vi "captureSpectImage.vi"(8 "error in (no error)":errorcluster, 9 "command_captureSpectImage":T1, 10 "model in":refnum<class "IModel.lvclass">, 11 "DefaultState in":refnum<class "DefaultState.lvclass">) -> (0 "error out":errorcluster, 2 "model out":refnum<class "IModel.lvclass">, 3 "DefaultState out":refnum<class "DefaultState.lvclass">)   [LabVIEW 2016, in "States.lvlib" / "DefaultState.lvclass"]
uses:
  DefaultState.lvclass
  IModel/IModel.lvclass
  ts_sallv_FiberSpectrograph/DataTypes/command_captureSpectImage.ctl
  Typedefs/CommandValue.ctl
  Typedefs/FiberSpectrographTypedefs.lvlib
  ts_sallv_FiberSpectrograph/SALLV_FiberSpectrograph.lvlib
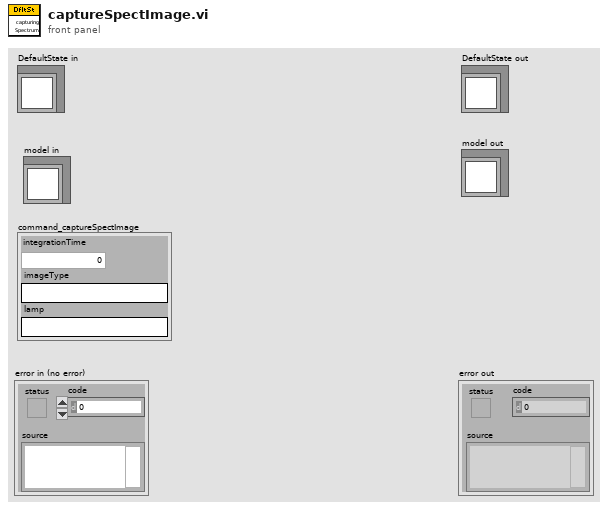
[diagram p1: front panel]
types:
  T1 = typedef "SALLV_FiberSpectrograph.lvlib/command_captureSpectImage.ctl" = cluster{"integrationTime":sgl, "imageType":string, "lamp":string}
  T2 = typedef "FiberSpectrographTypedefs.lvlib/CommandValue.ctl" = enum16{"clearError", "disable", "enable", "exit", "GoToStandby", "OnHeartbeat", "OnIncomingMessagingError", "OnInterrupt", "start", "captureSpectImage", "setSpectTempSetpoint", "stopImageCapture"}
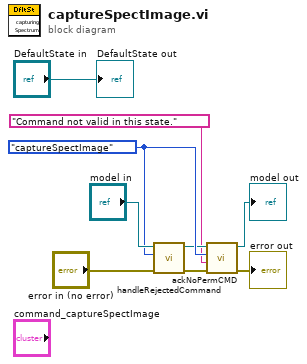
[diagram p0: block diagram]
diagram:
  w6 = CommandValue."captureSpectImage" ("CommandValue")
  n1 = call-dynamic "handleRejectedCommand.vi"("error in (no error)"="error in (no error)", "CommandValue"=w6, "IModel in"="model in") -> ("error out"=w3:errorcluster, "IModel out"=w5:refnum<class "IModel.lvclass">)  [unwired: 7 in]
  n2 = call-dynamic "ackNoPermCMD.vi"("error in (no error)"=w3, "rejectedReason"="Command not valid in this state.", "CommandValue"=w6, "IModel in"=w5) -> ("error out"=→"error out":errorcluster, "IModel out"=→"model out":refnum<class "IModel.lvclass">)  [unwired: 6 in]
  "DefaultState out" <- "DefaultState in"
